vi "Launch InstrumentStudio.vi"(11 "error in":errorcluster) -> (15 "error out":errorcluster)   [LabVIEW 2021, in "Converter.lvlib"]
uses:
  Converter.lvlib
  Path Functions/Path Functions.lvlib
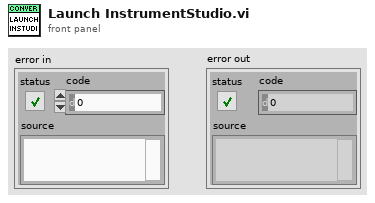
[diagram p1: front panel]
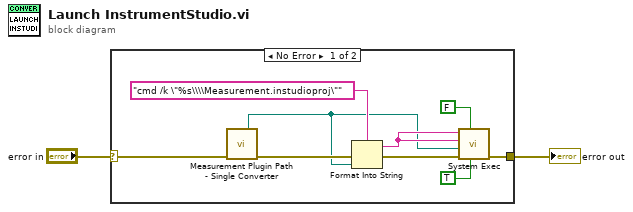
[diagram p0: block diagram]
diagram:
  n1 = case shown="No Error" "error in" {
    selector: "error in" -> [w10 w12]
    tunnel: [w6 w12] -> w2
    frame No Error {
      n2 = call "Measurement Plugin Path - Single Converter.vi"("error in"=w10) -> ("instrumentstudio folder"=w3:path, "error out"=w11:errorcluster)  [unwired: 2 in, 11 out]
      n3 = Format Into String(format string="cmd /k \"%s\\\\Measurement.instudioproj\"", error in=w11, w3) -> (resulting string=w5:string, error out=w9:errorcluster)  [unwired: 1 in]
      n4 = call <vilib>:"System Exec.vi"("run minimized? (F)"=TRUE, "wait until completion? (T)"=FALSE, "error in (no error)"=w9, "working directory"=w3, "standard input"=w5, "command line"=w5) -> ("error out"=w6:errorcluster)  [unwired: 2 in, 3 out]
    }
    frame Error {
    }
  }
  "error out" <- w2
